vi "Read_INI_File-Tracking_Val.vi"(8 "ERROR IN":errorcluster, 11 "[IN] refnum - ini file":T1) -> (0 "ERROR OUT":errorcluster, 1 "[OUT] Maximal angle":dbl, 3 "[OUT] Minimal length of a track":i32, 4 "[OUT] Minimal displacement":dbl, 5 "[OUT] Number of closing gaps":i32, 6 "[OUT] Maximal displacement":dbl, 7 "[OUT] Linearity":i32)   [LabVIEW 2017]
doc: "This subVI reads two values in the *ini file - under the \"Tracking Processing Values\" section"
uses:
  <vilib>/Utility/config.llb/Config Data RefNum.ctl
  <vilib>/Utility/config.llb/Read Key (I32).vi
  <vilib>/Utility/config.llb/Read Key (Double).vi
  <vilib>/Utility/config.llb/NI_LVConfig.lvlib
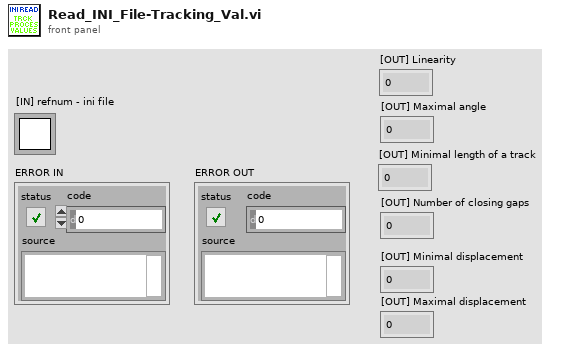
[diagram p1: front panel]
types:
  T1 = typedef "NI_LVConfig.lvlib/Config Data RefNum.ctl" = refnum<k1>
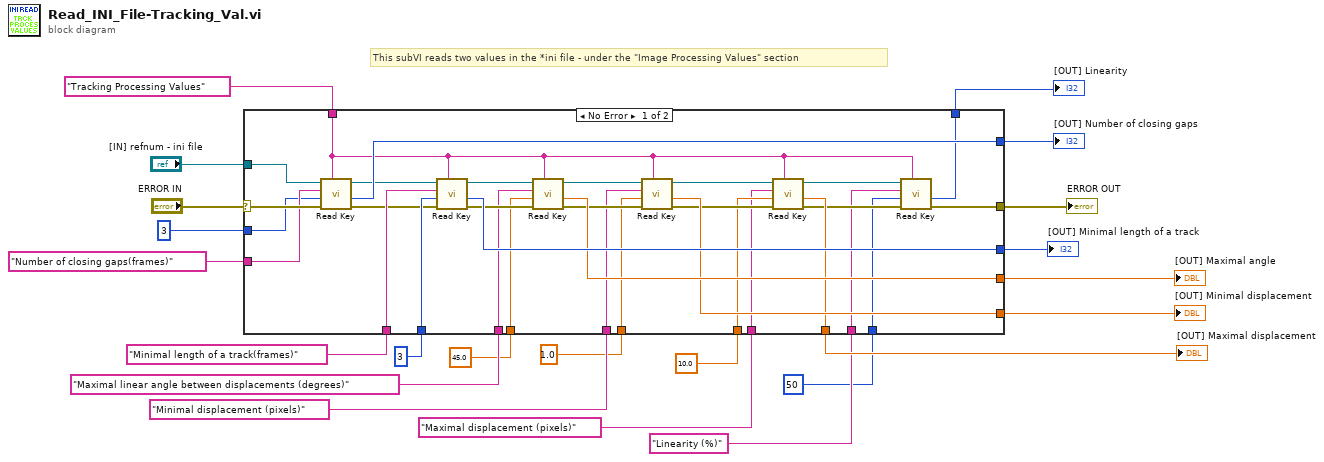
[diagram p0: block diagram]
diagram:
  # "This subVI reads two values in the *ini file - under the \"Image Processing Values\" section"
  n1 = case shown="No Error" "ERROR IN" {
    selector: "ERROR IN" -> [w54 w60]
    tunnel: "[IN] refnum - ini file" -> [w53 _]
    tunnel: "Tracking Processing Values" ("section") -> [w27 _]
    tunnel: "Number of closing gaps(frames)" ("key") -> [w52 _]
    tunnel: 3 ("default value") -> [w51 w61]
    tunnel: [w50 w61] -> w1
    tunnel: "Minimal length of a track(frames)" ("key") -> [w48 _]
    tunnel: 3 ("default value") -> [w47 w59]
    tunnel: [w25 w60] -> w15
    tunnel: [w45 w59] -> w14
    tunnel: "Maximal linear angle between displacements (degrees)" ("key") -> [w42 _]
    tunnel: 45.0 ("default value") -> [w41 w58]
    tunnel: [w40 w58] -> w11
    tunnel: "Minimal displacement (pixels)" ("key") -> [w37 _]
    tunnel: 1.0 ("default value") -> [w36 w57]
    tunnel: [w35 w57] -> w8
    tunnel: 10.0 ("default value") -> [w32 w56]
    tunnel: [w31 w56] -> w5
    tunnel: "Maximal displacement (pixels)" ("key") -> [w30 _]
    tunnel: "Linearity (%)" ("key") -> [w26 _]
    tunnel: 50 ("default value") -> [w24 w55]
    tunnel: [w23 w55] -> w2
    frame No Error {
      n2 = call-poly <vilib>:"Read Key.vi"("section"=w27, "error in (no error)"=w54, "default value"=w51, "key"=w52, "refnum"=w53) -> ("error out"=w46:errorcluster, "value"=w50:i32, "refnum out"=w49:T1)  [unwired: 3 in, 1 out]
      n3 = call-poly <vilib>:"Read Key.vi"("section"=w27, "error in (no error)"=w46, "default value"=w47, "key"=w48, "refnum"=w49) -> ("error out"=w43:errorcluster, "value"=w45:i32, "refnum out"=w44:T1)  [unwired: 3 in, 1 out]
      n4 = call-poly <vilib>:"Read Key.vi"("section"=w27, "error in (no error)"=w43, "default value"=w41, "key"=w42, "refnum"=w44) -> ("error out"=w38:errorcluster, "value"=w40:dbl, "refnum out"=w39:T1)  [unwired: 3 in, 1 out]
      n5 = call-poly <vilib>:"Read Key.vi"("section"=w27, "error in (no error)"=w38, "default value"=w36, "key"=w37, "refnum"=w39) -> ("error out"=w33:errorcluster, "value"=w35:dbl, "refnum out"=w34:T1)  [unwired: 3 in, 1 out]
      n6 = call-poly <vilib>:"Read Key.vi"("section"=w27, "error in (no error)"=w33, "default value"=w32, "key"=w30, "refnum"=w34) -> ("error out"=w28:errorcluster, "value"=w31:dbl, "refnum out"=w29:T1)  [unwired: 3 in, 1 out]
      n7 = call-poly <vilib>:"Read Key.vi"("section"=w27, "error in (no error)"=w28, "default value"=w24, "key"=w26, "refnum"=w29) -> ("error out"=w25:errorcluster, "value"=w23:i32)  [unwired: 3 in, 2 out]
    }
    frame Error {
    }
  }
  "ERROR OUT" <- w15
  "[OUT] Number of closing gaps" <- w1
  "[OUT] Minimal length of a track" <- w14
  "[OUT] Maximal angle" <- w11
  "[OUT] Minimal displacement" <- w8
  "[OUT] Maximal displacement" <- w5
  "[OUT] Linearity" <- w2
